vi "Load_from_DB_subVin.vi"(8 "error in (no error)":errorcluster, 10 "Wybranie bazy danych - plik .UDL":path, 11 "Wybranie tabeli z bazy danych":string) -> (0 "error out":errorcluster)   [LabVIEW 2019]
doc: "This Vi provides data to be loaded from DB. The input is source - Data Base path, .UDL file, Table name - we need to know from which table we want to load from. This Vi don't parametrize other select options, so this load like \" Select * from /table_name/.\nThe last input is error in. The outputs are the data recieved and error out."
uses:
  <vilib>/addons/database/Connection.llb/DB Tools Open Connec (Path).vi
  <vilib>/addons/database/NI_Database_API.lvlib
panel:
  out "Table Data":string[][](table)
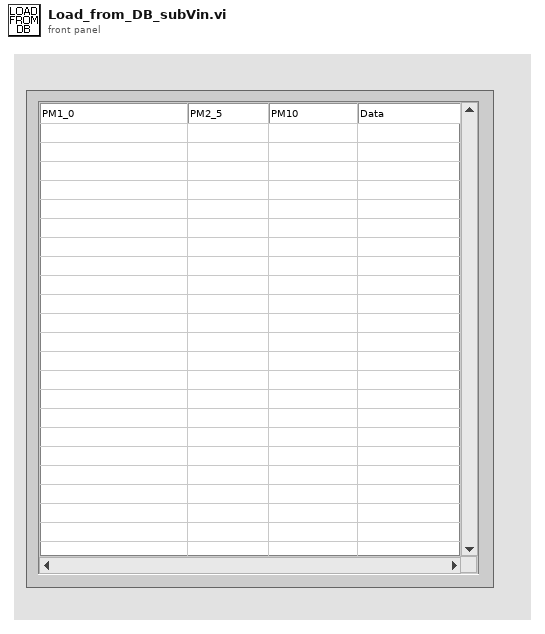
[diagram p1: front panel]
types:
  T1 = typedef "NI_Database_API.lvlib/Conn ObjectReference.ctl" = refnum<k1>
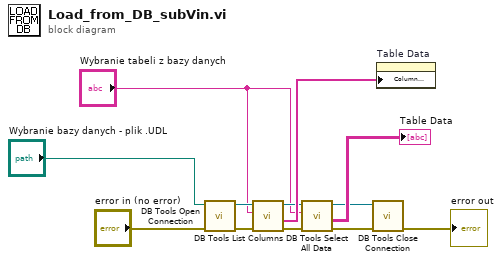
[diagram p0: block diagram]
diagram:
  n1 = call-poly <vilib>:"DB Tools Open Connection.vi"("error in (no error)"="error in (no error)", "connection information"="Wybranie bazy danych - plik .UDL") -> ("error out"=w7:errorcluster, "connection reference"=w10:T1)  [unwired: 6 in]
  n2 = call <vilib>:"DB Tools List Columns.vi"("error in (no error)"=w7, "table"="Wybranie tabeli z bazy danych", "connection reference"=w10) -> ("error out"=w6:errorcluster, "columns"=w9:string[], "connection reference out"=w8:T1)  [unwired: 1 in, 1 out]
  n3 = call <vilib>:"DB Tools Select All Data.vi"("error in (no error)"=w6, "table"="Wybranie tabeli z bazy danych", "connection reference"=w8) -> ("error out"=w2:errorcluster, "data"=→"Table Data":string[][], "connection reference out"=w3:T1)  [unwired: 3 in]
  n4 = call <vilib>:"DB Tools Close Connection.vi"("error in (no error)"=w2, "connection reference"=w3) -> ("error out"=→"error out":errorcluster)  [unwired: 5 in]
  n5 = property on="Table Data" class="Tbl (strict)"("Column Headers[]"=w9) -> ()  [unwired: 2 in, 2 out]
